vi "DEV Check Column Clusters.vi"(8 "Error In":errorcluster) -> (0 "Error Out":errorcluster, 3 "Results":cluster{"Cluster matches DB?":bool[]}[](array[cluster]))   [LabVIEW 2018, in "Database.lvlib"]
uses:
  Database.lvlib
  Items--cluster.ctl
  Purchased_Items--cluster.ctl
  Visits--cluster.ctl
panel:
  in  "Visits":T1 {"TotalSpend" format="£%.2g"; "SpendTaxedA" format="£%.2g"; "SpendTaxedB" format="£%.2g"}
  in  "Purchased_Items":T2 {"TotalPriceIncludingDiscount" format="£%.2g"; "TotalDiscount" format="£%.2g"}
  in  "Items":T3
  # "Idea: Purchased Items doesn't need Date because can join with Visit ID"
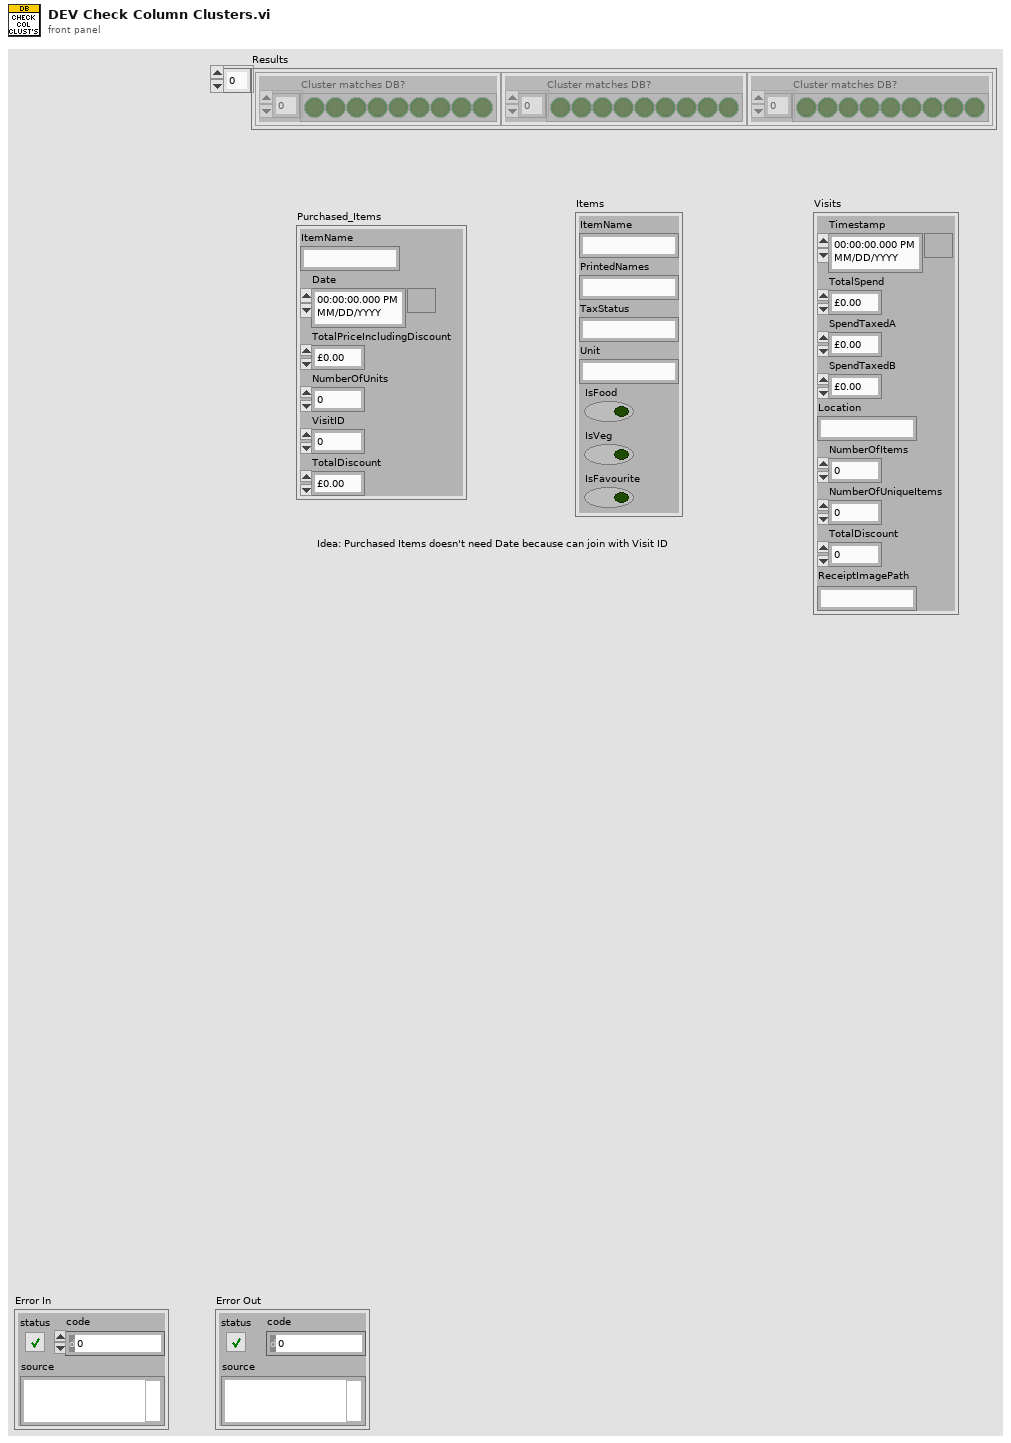
[diagram p1: front panel]
types:
  T1 = typedef "Database.lvlib/Visits--cluster.ctl" = cluster{"Timestamp":timestamp, "TotalSpend":dbl, "SpendTaxedA":dbl, "SpendTaxedB":dbl, "Location":string, "NumberOfItems":i32, "NumberOfUniqueItems":i32, "TotalDiscount":dbl, "ReceiptImagePath":string}
  T2 = typedef "Database.lvlib/Purchased_Items--cluster.ctl" = cluster{"ItemName":string, "Date":timestamp, "TotalPriceIncludingDiscount":dbl, "NumberOfUnits":i32, "VisitID":i32, "TotalDiscount":dbl}
  T3 = typedef "Database.lvlib/Items--cluster.ctl" = cluster{"ItemName":string, "PrintedNames":string, "TaxStatus":string, "Unit":string, "IsFood":bool, "IsVeg":bool, "IsFavourite":bool}
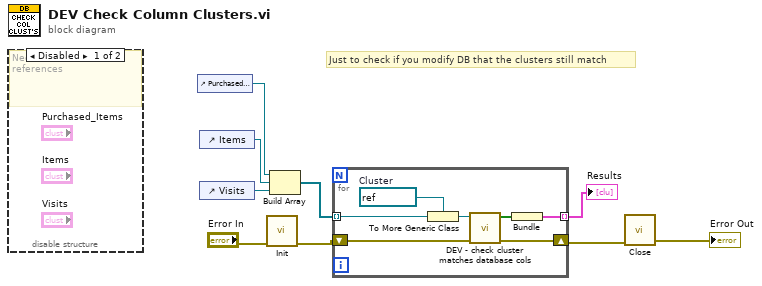
[diagram p0: block diagram]
diagram:
  # "Just to check if you modify DB that the clusters still match"
  n1 = disable-structure shown="Disabled" {
    frame Disabled {
      # "Need controls to make references"
    }
    frame Enabled {
    }
  }
  n2 = control-ref of="Purchased_Items"() -> (w5:refnum<vi>)
  n3 = control-ref of="Items"() -> (w6:refnum<vi>)
  n4 = control-ref of="Visits"() -> (w7:refnum<vi>)
  n5 = call "Init.vi"("Error In"="Error In") -> ("Error Out"=w4:errorcluster)  [unwired: 10 in]
  n6 = Build Array(w5, w6, w7) -> (w9:refnum<vi>[])
  n7 = for {
    shift-right: [w15] -> w1
    shift-left: w4 -> [w16]
    tunnel: [w11] -> w8 mode=indexing
    tunnel: w9 -> [w10] mode=indexing
    w14 = refnum<vi> refnum  # Cluster
    n8 = To More Generic Class(target class=w14, reference=w10) -> (generic class reference=w13:refnum<vi>)
    n9 = call "DEV - check cluster matches database cols.vi"("Error In"=w16, "Generic Cluster Reference"=w13) -> ("Error Out"=w15:errorcluster, "Cluster matches DB?"=w12:bool[])  [unwired: 8 in]
    n10 = Bundle("Cluster matches DB?"=w12) -> (w11:cluster{"Cluster matches DB?":bool[]})  [unwired: 1 in]
  }
  "Results" <- w8
  n11 = call "Close.vi"("Error In"=w1) -> ("Error Out"=→"Error Out":errorcluster)  [unwired: 10 in]
